vi "createTelemetry.vi"(8 "error in (no error)":errorcluster, 11 "Boot in":refnum<class "Boot.lvclass">) -> (0 "error out":errorcluster, 2 "Telemetry":refnum<class "Telemetry.lvclass">, 3 "Boot out":refnum<class "Boot.lvclass">)   [LabVIEW 2016, in "Boot.lvclass"]
uses:
  Boot.lvclass
  Telemetry/Telemetry.lvclass
  Boot.lvclass/Boot.ctl
  Telemetry/Telemetry.lvclass/Telemetry.ctl
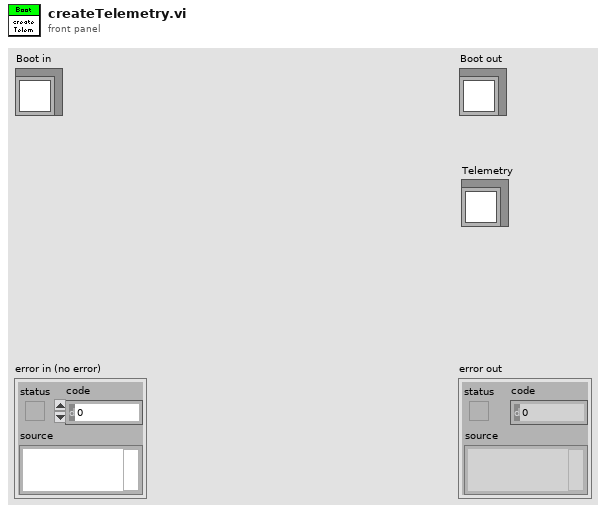
[diagram p1: front panel]
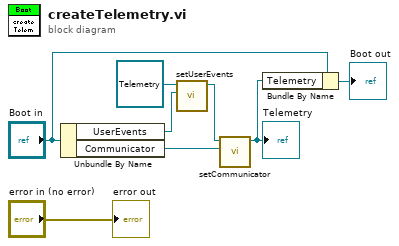
[diagram p0: block diagram]
diagram:
  n1 = Unbundle By Name("Boot in") -> ("UserEvents"=w2:refnum<class "UserEvents.lvclass">, "Communicator"=w1:refnum<class "Communicator.lvclass">)
  n2 = call "setUserEvents.vi"("UserEvents"=w2, "Telemetry in"=refnum<class "Telemetry.lvclass"> refnum ("Telemetry.lvclass")) -> ("Telemetry out"=w5:refnum<class "Telemetry.lvclass">)  [unwired: 9 in]
  n3 = call "setCommunicator.vi"("Communicator"=w1, "Telemetry in"=w5) -> ("Telemetry out"=w4:refnum<class "Telemetry.lvclass">)  [unwired: 9 in]
  "Telemetry" <- w4
  n4 = Bundle By Name(cluster="Boot in", "Telemetry"=w4) -> (→"Boot out":refnum<class "Boot.lvclass">)
  "error out" <- "error in (no error)"
